vi "單軸復歸.vi"(8 "stop":bool, 11 "Axis_ID":i32) -> ()   [LabVIEW 2015]
uses:
  <userlib>/ADLINK/APS168.lvlib
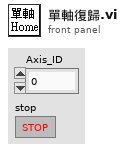
[diagram p1: front panel]
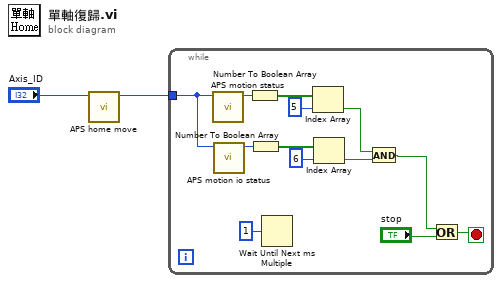
[diagram p0: block diagram]
diagram:
  n1 = call <userlib>:"APS home move.vi"("Axis_ID"="Axis_ID") -> ("function return"=w2:i32)  [unwired: 9 in, 1 out]
  n2 = while {
    tunnel: w2 -> [w9]
    stop <- w6 stop-if-true
    n3 = call <userlib>:"APS motion status.vi"("Axis_ID"=w9) -> ("function return"=w15:i32)  [unwired: 9 in, 1 out]
    n4 = call <userlib>:"APS motion io status.vi"("Axis_ID"=w9) -> ("function return"=w10:i32)  [unwired: 9 in, 1 out]
    n5 = Number To Boolean Array(number=w15) -> (Boolean array=w14:bool[])
    n6 = Number To Boolean Array(number=w10) -> (Boolean array=w11:bool[])
    n7 = Wait Until Next ms Multiple(millisecond multiple=u32 1) -> ()  [unwired: 1 out]
    n8 = Index Array(array=w14, index=5 ("索引")) -> (element=w8:bool)
    n9 = Index Array(array=w11, index=6 ("索引")) -> (element=w7:bool)
    n10 = And(x=w8, y=w7) -> (x .and. y?=w4:bool)
    n11 = Or(x=w4, y="stop") -> (x .or. y?=w6:bool)
  }
